vi "标样核查操作框.vi"() -> ()   [LabVIEW 2016, in "main.lvlib"]
uses:
  main.lvlib
  <vilib>/LAVA/UI Tools/Dialog/Dialog/Dialog/Dialog__lava_lib_ui_tools.lvclass
  EXO2/EXO2.lvlib
  NAQ_DO/NAQ_DO.lvlib
  bbe/bbe.lvlib
  DAM395CF/PLC.lvlib
panel:
  out "保存标样":bool=TRUE
  in  "保存水样值":bool
  in  "仪器测试":bool
  out "仪器通讯":bool
  in  "保存标样值":bool
  in  "标准值":dbl
  out "测量值":dbl
  in  "核查参数":u16(ring) items=["水温", "电导率", "浊度", "pH", "溶解氧", "叶绿素a"]
  # "标样核查"
  # "操作说明：\n1、点击仪器测试\n2、观察通讯指示灯，亮起后，可进行下一步操作\n3、选择核查参数\n4、输入标准值\n5、待测试值稳定后，点击保存标样核查\n6、结束"
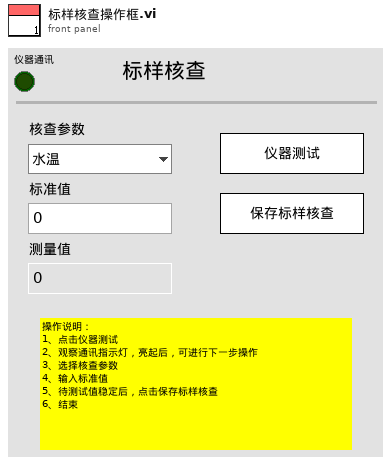
[diagram p1: front panel]
types:
  T1 = typedef "剖面数据_EXO2.ctl" = cluster{"时间":timestamp, "测量模式":string, "数据类型":string, "数据标识":string, "湖面水深":sgl, "缆绳下放长度":sgl, "层数":u16, "row":u16, "水温":sgl, "比电导率":sgl, "电导率":sgl, "盐度":sgl, "总溶解固体":sgl, "pH":sgl, "pHmV":sgl, "ORP":sgl, "饱和度":sgl, "DO":sgl, "浊度":sgl, "叶绿素a":sgl, "水深":sgl, "设置水深":sgl}
  T2 = typedef "剖面数据_bbe_NAQDO.ctl" = cluster{"时间":timestamp, "测量模式":string, "数据类型":string, "数据标识":string, "湖面水深":sgl, "缆绳下放长度":sgl, "层数":u16, "row":u16, "水温":sgl, "DO":sgl, "饱和度":sgl, "绿藻":sgl, "蓝藻":sgl, "硅甲藻":sgl, "隐藻":sgl, "黄色物质":sgl, "总藻":sgl, "透光率":sgl, "水深":sgl, "设置水深":sgl}
  T3 = enum16{"open", "poll", "close", "run", "stop", "shutdown"}
  T4 = cluster{"Time":timestamp, "Temp":dbl, "SpCond":dbl, "Cond":dbl, "Sal":dbl, "TDS":dbl, "pH":dbl, "pH mV":dbl, "orp":dbl, "ODO %":dbl, "ODO mg/L":dbl, "Turb":dbl, "Chl":dbl, "Depth":dbl}
  T5 = cluster{"时间标识":timestamp, "DO [mg/L]":dbl, "DO [%]":dbl}
  T6 = typedef "集成多参数单参数字段定义.ctl" = cluster{"时间":timestamp, "测量模式":string, "数据类型":string, "检测值":sgl, "单位":string, "数据标识":string, "信号值":sgl, "标样参考值":sgl, "因子编码":string, "探头温度":sgl, "LastTime":timestamp}
  T7 = cluster{"时间":timestamp, "Temp [℃]":dbl, "Green Algae [μg/L]":dbl, "Bluegreen [μg/L]":dbl, "Diatoms [μg/L]":dbl, "Cryptophyta [μg/L]":dbl, "Yellow substances [r.u.]":dbl, "Total Conc [μg/L]":dbl, "Transmission [%]":dbl, "Depth [m]":dbl}
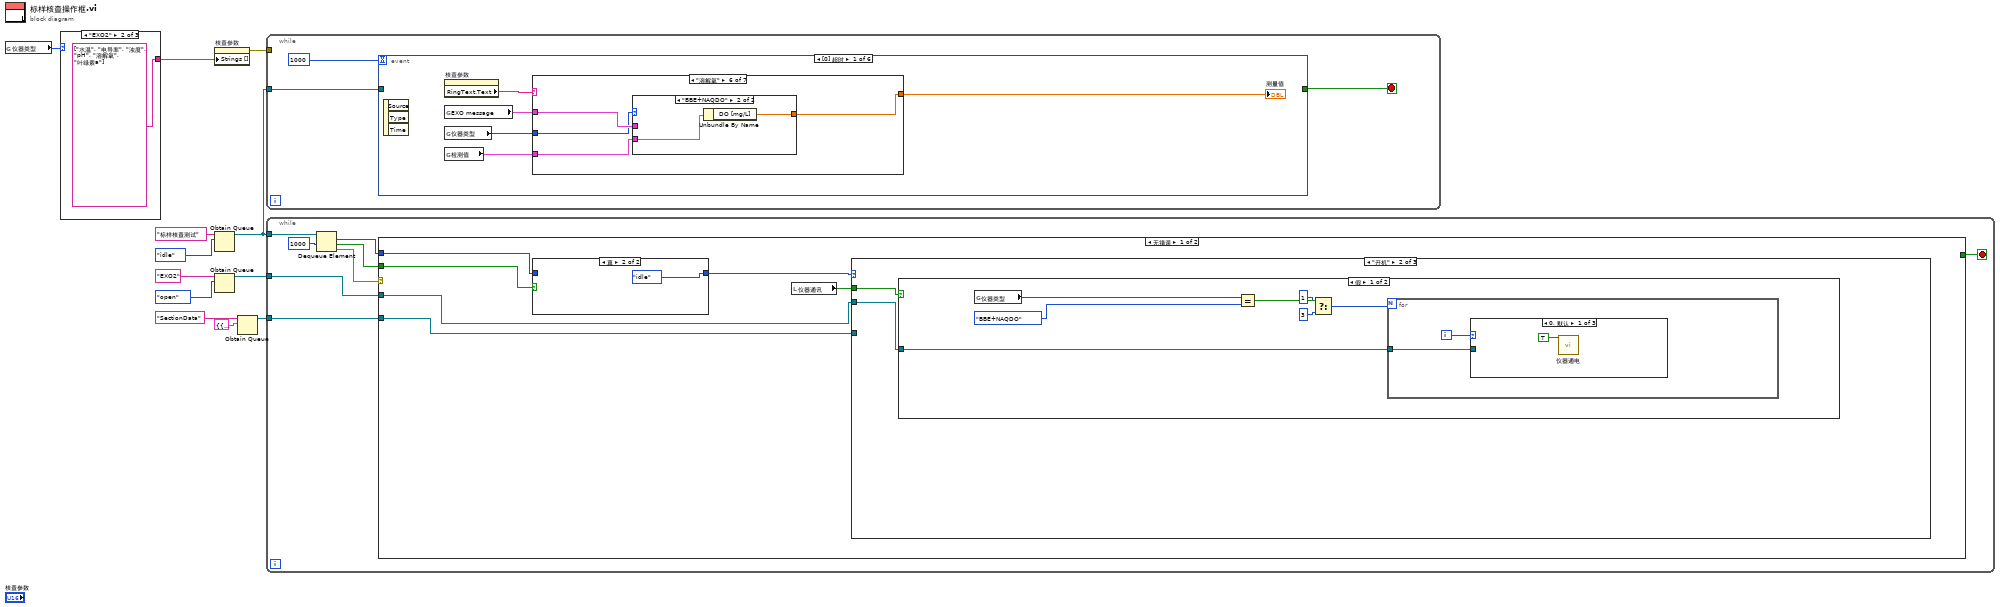
[diagram p0: block diagram]
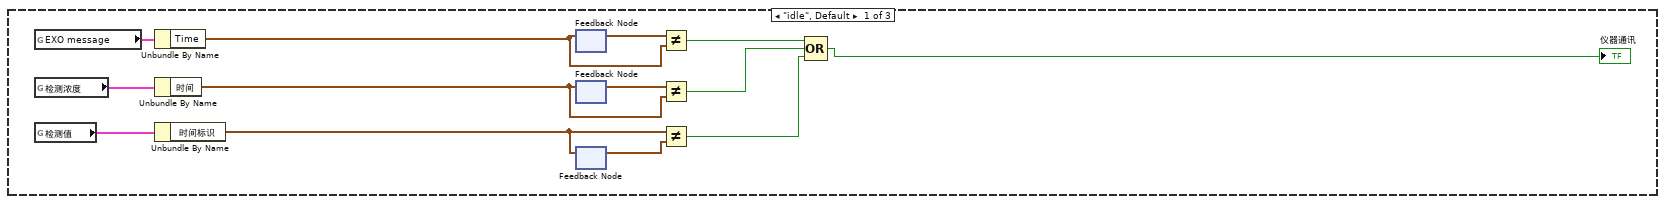
[diagram p2: hidden frame]
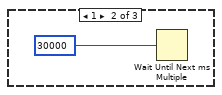
[diagram p3: hidden frame]
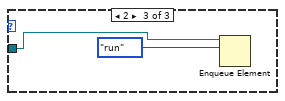
[diagram p4: hidden frame]
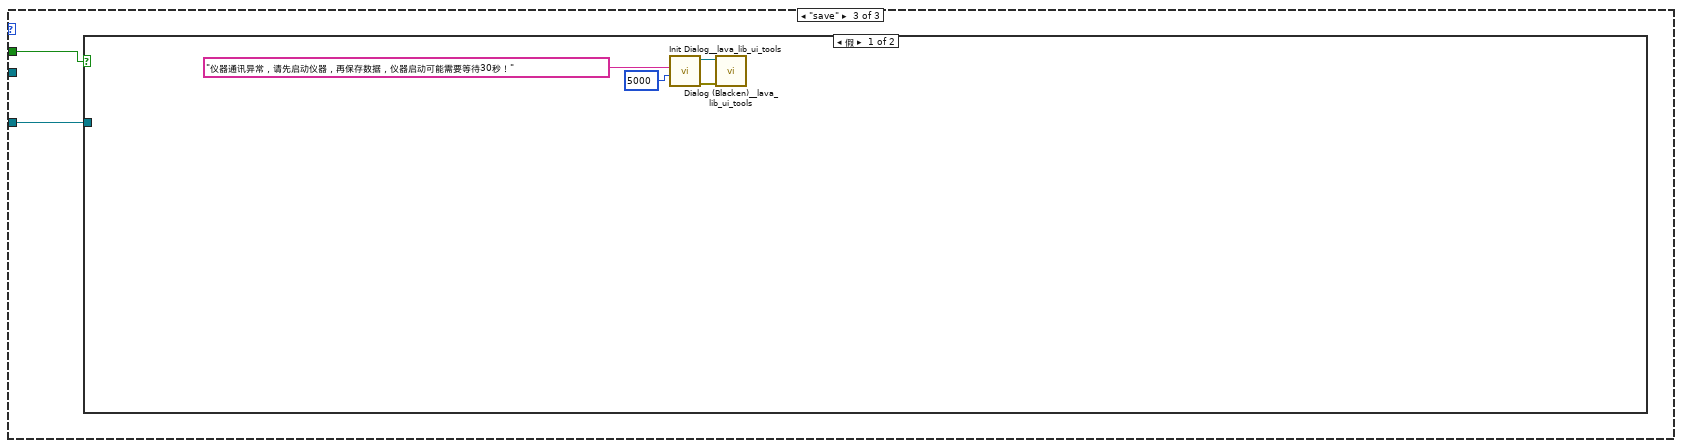
[diagram p6: hidden frame]
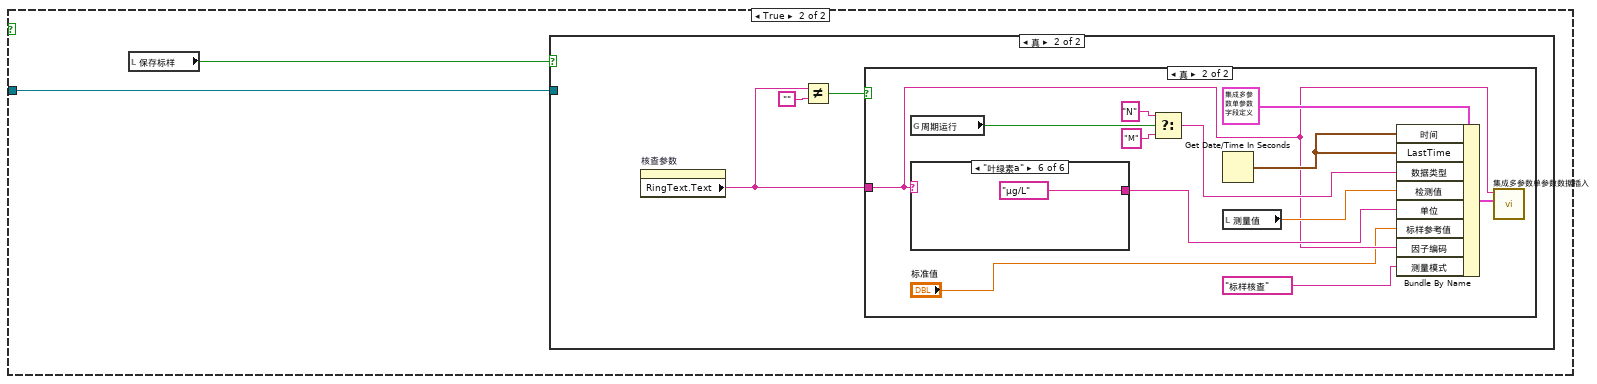
[diagram p7: hidden frame]
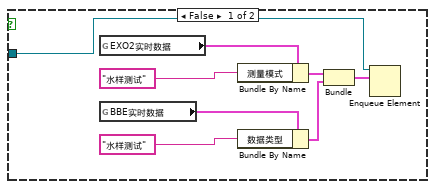
[diagram p8: hidden frame]
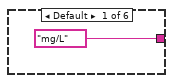
[diagram p10: hidden frame]
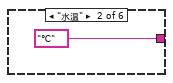
[diagram p11: hidden frame]
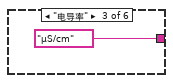
[diagram p12: hidden frame]
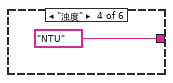
[diagram p13: hidden frame]
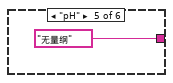
[diagram p14: hidden frame]
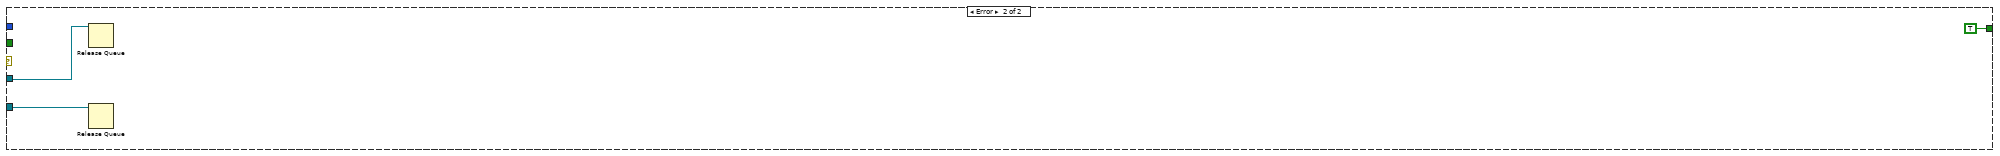
[diagram p16: hidden frame]
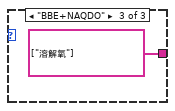
[diagram p18: hidden frame]
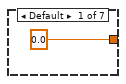
[diagram p19: hidden frame]
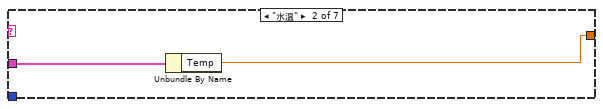
[diagram p20: hidden frame]
diagram:
  n1 = global read "全局断电保存变量.vi" "仪器类型"() -> (w12:enum16{"EXO2", "BBE+NAQDO"})
  n2 = case shown="\"EXO2\"" w12 {
    tunnel: [_ string[] ["水温", "电导率", "浊度", "pH", "溶解氧", "叶绿素a"] string[] ["溶解氧"]] -> w11
    frame Default {
    }
    frame "EXO2" {
    }
    frame "BBE+NAQDO" {
    }
  }
  n3 = property on="核查参数" class="Ring (严格)"("Strings []"=w11) -> (error out=w10:errorcluster)  [unwired: 2 in, 1 out]
  n4 = Obtain Queue(name (unnamed)="标样核查测试" ("名称（未命名）"), element data type=enum16{"idle", "开机", "save"}."idle" ("枚举")) -> (queue out=w7:refnum<queue>)  [unwired: 3 in, 2 out]
  n5 = Obtain Queue(name (unnamed)="EXO2" ("名称（未命名）"), element data type=T3."open" ("枚举")) -> (queue out=w4:refnum<queue>)  [unwired: 3 in, 2 out]
  n6 = Obtain Queue(name (unnamed)="SectionData" ("名称（未命名）"), element data type=cluster{"EXO2 message":T1, "bbe message":T2} {"EXO2 message"={"时间"=timestamp(0 s since 1904-01-01), "测量模式"="水样测试", "数据类型"="N", "数据标识"="N", "湖面水深"=0.0, "缆绳下放长度"=0.0, "层数"=0, "row"=0, "水温"=0.0, "比电导率"=0.0, "电导率"=0.0, "盐度"=0.0, "总溶解固体"=0.0, "pH"=0.0, "pHmV"=0.0, "ORP"=0.0, "饱和度"=0.0, "DO"=0.0, "浊度"=0.0, "叶绿素a"=0.0, "水深"=0.0, "设置水深"=0.0}, "bbe message"={"时间"=timestamp(0 s since 1904-01-01), "测量模式"="水样测试", "数据类型"="N", "数据标识"="N", "湖面水深"=0.0, "缆绳下放长度"=0.0, "层数"=0, "row"=0, "水温"=0.0, "DO"=0.0, "饱和度"=0.0, "绿藻"=0.0, "蓝藻"=0.0, "硅甲藻"=0.0, "隐藻"=0.0, "黄色物质"=0.0, "总藻"=0.0, "透光率"=0.0, "水深"=0.0, "设置水深"=0.0}} ("簇")) -> (queue out=w1:refnum<queue>)  [unwired: 3 in, 2 out]
  n7 = while {
    tunnel: w10 -> [_]
    tunnel: w7 -> [w15]
    stop <- w17 stop-if-true
    n8 = event shown="[0] 超时" {
      selector: _ -> [_ _ _ _ _ _]
      dyn-events: _ -> [_ _ _ _ _ _]
      timeout: 1000 -> [_ _ _ _ _ _]
      tunnel: [_ _ _ _ TRUE _] -> w17
      tunnel: w15 -> [_ w42 w46 w51 w52 _]
      event Timeout {
        n9 = event-data() -> ()  [unwired: 1 in, 3 out]
        n10 = property on="核查参数" class="Ring (严格)"() -> ("RingText.Text"=w22:string)  [unwired: 2 in, 2 out]
        n11 = global read "EXO2全局变量.vi" "EXO message"() -> (w20:T4)
        n12 = global read "全局断电保存变量.vi" "仪器类型"() -> (w19:enum16{"EXO2", "BBE+NAQDO"})
        n13 = global read "过程变量.vi" "检测值"() -> (w21:T5)
        n14 = case shown="\"溶解氧\"" w22 {
          tunnel: w21 -> [_ _ _ _ _ w32 _]
          tunnel: w20 -> [_ w25 w27 w29 w31 w35 w41]
          tunnel: w19 -> [_ _ _ _ _ w33 _]
          tunnel: [0.0 ("ODO mg/L") w24 w26 w28 w30 w34 w40] -> w18
          frame Default {
          }
          frame "水温" {
            n15 = Unbundle By Name(w25) -> ("Temp"=w24:dbl)
          }
          frame "电导率" {
            n16 = Unbundle By Name(w27) -> ("SpCond"=w26:dbl)
          }
          frame "浊度" {
            n17 = Unbundle By Name(w29) -> ("Turb"=w28:dbl)
          }
          frame "pH" {
            n18 = Unbundle By Name(w31) -> ("pH"=w30:dbl)
          }
          frame "溶解氧" {
            n19 = case shown="\"BBE+NAQDO\"" w33 {
              tunnel: w35 -> [w37 _]
              tunnel: [w36 w38] -> w34
              tunnel: w32 -> [_ w39]
              frame "EXO2", Default {
                n20 = Unbundle By Name(w37) -> ("ODO mg/L"=w36:dbl)
              }
              frame "BBE+NAQDO" {
                n21 = Unbundle By Name(w39) -> ("DO [mg/L]"=w38:dbl)
              }
            }
          }
          frame "叶绿素a" {
            n22 = Unbundle By Name(w41) -> ("ODO mg/L"=w40:dbl)
          }
        }
        "测量值" <- w18
      }
      event "保存标样值": Value Change {
        n23 = event-data() -> ()  [unwired: 1 in, 6 out]
        n24 = flat-sequence {
          tunnel: w42 -> [w45]
          frame #0 {
            "保存标样" <- TRUE ("保存标样")
          }
          frame #1 {
            n25 = Enqueue Element(queue=w45, element=enum16{"idle", "开机", "save"}."save" ("元素")) -> ()  [unwired: 2 in, 3 out]
          }
        }
      }
      event "保存水样值": Value Change {
        n26 = event-data() -> ()  [unwired: 1 in, 6 out]
        n27 = flat-sequence {
          tunnel: w46 -> [w49]
          frame #0 {
            n28 = local write "保存标样"(FALSE ("保存标样")) -> ()
          }
          frame #1 {
            n29 = Enqueue Element(queue=w49, element=enum16{"idle", "开机", "save"}."save" ("元素")) -> ()  [unwired: 2 in, 3 out]
          }
        }
      }
      event "仪器测试": Value Change {
        n30 = event-data() -> ()  [unwired: 1 in, 1 out]
        n31 = Enqueue Element(queue=w51, element=enum16{"idle", "开机", "save"}."开机" ("元素")) -> ()  [unwired: 2 in, 3 out]
      }
      event Panel Close {
        n32 = event-data() -> ()  [unwired: 1 in, 4 out]
        n33 = Release Queue(queue=w52) -> ()  [unwired: 2 in, 3 out]
      }
      event "标准值": Mouse Down {
        n34 = event-data() -> ("CtlRef"=w57:refnum<vi>)  [unwired: 1 in]
        n35 = property class="DigNum (严格)"(reference=w57) -> (reference out=w54:refnum<vi>, "Value"=w56:dbl)  [unwired: 1 in, 1 out]
        n36 = call "数字键盘.vi"("OldNumber"=w56) -> ("NewNumber"=w55:dbl)
        n37 = property class="DigNum (严格)"(reference=w54, "Value"=w55) -> ()  [unwired: 1 in, 2 out]
      }
    }
  }
  n38 = while {
    tunnel: w7 -> [w65]
    tunnel: w4 -> [w62]
    tunnel: w1 -> [w58]
    stop <- w60 stop-if-true
    n39 = Dequeue Element(queue=w65, timeout in ms (-1)=1000 ("超时毫秒(-1)")) -> (element=w63:enum16{"idle", "开机", "save"}, timed out?=w64:bool, error out=w61:errorcluster)  [unwired: 1 in, 1 out]
    n40 = case shown="无错误" w61 {
      tunnel: w64 -> [w71 _]
      tunnel: w63 -> [w70 _]
      tunnel: w62 -> [w68 w140]
      tunnel: [_ TRUE] -> w60
      tunnel: w58 -> [w67 w139]
      frame No Error {
        n41 = case shown="真" w71 {
          tunnel: w70 -> [w137 _]
          tunnel: [w137 enum16{"idle", "开机", "save"}."idle" ("枚举")] -> w69
          frame False {
          }
          frame True {
          }
        }
        n42 = local read "仪器通讯"() -> (w66:bool)
        n43 = case shown="\"开机\"" w69 {
          tunnel: w68 -> [_ w86 _]
          tunnel: w67 -> [_ _ w101]
          tunnel: w66 -> [_ w85 w100]
          frame "idle", Default {
            n44 = global read "EXO2全局变量.vi" "EXO message"() -> (w84:T4)
            n45 = global read "过程变量.vi" "检测浓度"() -> (w83:T7)
            n46 = global read "过程变量.vi" "检测值"() -> (w82:T5)
            n47 = Unbundle By Name(w84) -> ("Time"=w80:timestamp)
            n48 = Unbundle By Name(w83) -> ("时间"=w78:timestamp)
            n49 = Unbundle By Name(w82) -> ("时间标识"=w77:timestamp)
            n50 = feedback-in #1(w80) -> ()
            n51 = feedback #1() -> (w81:timestamp)  [unwired: 1 in]
            n52 = feedback #2() -> (w79:timestamp)  [unwired: 1 in]
            n53 = feedback-in #2(w78) -> ()
            n54 = feedback #3() -> (w76:timestamp)  [unwired: 1 in]
            n55 = feedback-in #3(w77) -> ()
            n56 = Not Equal?(x=w81, y=w80) -> (x != y?=w75:bool)
            n57 = Not Equal?(x=w79, y=w78) -> (x != y?=w74:bool)
            n58 = Not Equal?(x=w77, y=w76) -> (x != y?=w73:bool)
            n59 = Compound Arithmetic op=OR ("复合运算")(w75, w74, w73) -> (→"仪器通讯":bool)
          }
          frame "开机" {
            n60 = case shown="假" w85 {
              tunnel: w86 -> [w93 _]
              frame False {
                n61 = global read "全局断电保存变量.vi" "仪器类型"() -> (w92:enum16{"EXO2", "BBE+NAQDO"})
                n62 = Equal?(x=w92, y=enum16{"EXO2", "BBE+NAQDO"}."BBE+NAQDO") -> (x = y?=w90:bool)
                n63 = Select(t=1, s=w90, f=3) -> (s? t:f=w87:i32)
                n64 = for {
                  N: w87 -> [_]
                  tunnel: w93 -> [w94]
                  i -> [w95]
                  n65 = case shown="0, 默认" w95 {
                    tunnel: w94 -> [_ _ w98]
                    frame 0, Default {
                      n66 = call "仪器通电.vi"("value"=TRUE) -> ()  [unwired: 10 in, 1 out]
                    }
                    frame 1 {
                      n67 = Wait Until Next ms Multiple(millisecond multiple=u32 30000 ("毫秒倍数")) -> ()  [unwired: 1 out]
                    }
                    frame 2 {
                      n68 = Enqueue Element(queue=w98, element=T3."run" ("元素")) -> ()  [unwired: 2 in, 3 out]
                    }
                  }
                }
              }
              frame True {
              }
            }
          }
          frame "save" {
            n69 = case shown="假" w100 {
              tunnel: w101 -> [_ w106]
              frame False {
                n70 = call <vilib>:"Init Dialog__lava_lib_ui_tools.vi"("Timeout (-1)"=5000, "Message"="仪器通讯异常，请先启动仪器，再保存数据，仪器启动可能需要等待30秒！") -> ("error out"=w104:errorcluster, "Dialog out"=w103:refnum<class "Dialog__lava_lib_ui_tools.lvclass">)  [unwired: 8 in]
                n71 = call-dynamic "Dialog (Blacken)__lava_lib_ui_tools.vi"("error in (no error)"=w104, "Dialog in"=w103) -> ()  [unwired: 6 in, 4 out]
              }
              frame True {
                n72 = local read "保存标样"() -> (w107:bool)
                n73 = case shown="真" w107 {
                  tunnel: w106 -> [w108 _]
                  frame False {
                    n74 = global read "全局非断电保持变量.vi" "EXO2实时数据"() -> (w115:T1)
                    n75 = global read "全局非断电保持变量.vi" "BBE实时数据"() -> (w114:T2)
                    n76 = Bundle By Name(cluster=w115, "测量模式"="水样测试" ("数据类型")) -> (w112:T1)
                    n77 = Bundle By Name(cluster=w114, "数据类型"="水样测试") -> (w111:T2)
                    n78 = Bundle("EXO2实时数据"=w112, "BBE实时数据"=w111) -> (w113:cluster{"EXO2实时数据":T1, "BBE实时数据":T2})  [unwired: 1 in]
                    n79 = Enqueue Element(queue=w108, element=w113) -> ()  [unwired: 2 in, 3 out]
                  }
                  frame True {
                    n80 = property on="核查参数" class="Ring (严格)"() -> ("RingText.Text"=w118:string)  [unwired: 2 in, 2 out]
                    n81 = Not Equal?(x=w118, y="") -> (x != y?=w116:bool)
                    n82 = case shown="真" w116 {
                      tunnel: w118 -> [_ w121]
                      frame False {
                      }
                      frame True {
                        n83 = global read "全局断电保存变量.vi" "周期运行"() -> (w126:bool)
                        n84 = case shown="\"叶绿素a\"" w121 {
                          tunnel: ["mg/L" ("单位") "℃" ("单位") "μS/cm" ("单位") "NTU" ("单位") "无量纲" ("单位") "μg/L" ("单位")] -> w123
                          frame Default {
                          }
                          frame "水温" {
                          }
                          frame "电导率" {
                          }
                          frame "浊度" {
                          }
                          frame "pH" {
                          }
                          frame "叶绿素a" {
                          }
                        }
                        n85 = Select(t="N" ("数据类型"), s=w126, f="M" ("数据类型")) -> (s? t:f=w125:string)
                        n86 = Get Date/Time In Seconds() -> (seconds since 1Jan1904=w124:timestamp)
                        n87 = local read "测量值"() -> (w122:dbl)
                        n88 = Bundle By Name(cluster=T6 {"时间"=timestamp(0 s since 1904-01-01), "测量模式"="标样核查", "数据类型"="N", "检测值"=0.0, "单位"="mg/L", "数据标识"="N", "信号值"=0.0, "标样参考值"=0.0, "因子编码"="", "探头温度"=0.0, "LastTime"=timestamp(0 s since 1904-01-01)} ("data"), "时间"=w124, "LastTime"=w124, "数据类型"=w125, "检测值"=w122, "单位"=w123, "标样参考值"="标准值", "因子编码"=w121, "测量模式"="标样核查") -> (w129:T6)
                        n89 = call "集成多参数单参数数据插入.vi"("Tabe Name"=w121, "data"=w129) -> ()  [unwired: 8 in, 1 out]
                      }
                    }
                  }
                }
              }
            }
          }
        }
      }
      frame Error {
        n90 = Release Queue(queue=w140) -> ()  [unwired: 2 in, 3 out]
        n91 = Release Queue(queue=w139) -> ()  [unwired: 2 in, 3 out]
      }
    }
  }
